vi "PXI-Tasks to Channel Names.vi"(1 "Array":T1[](array[typedef])) -> (0 "Channel Names":string[](array[string]))   [LabVIEW 2020]
uses:
  Type Defs/Task Struct.ctl
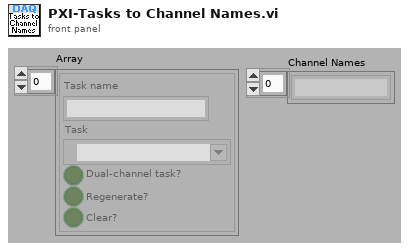
[diagram p1: front panel]
types:
  T1 = typedef "Task Struct.ctl" = cluster{"Task name":string, "Task":refnum<k21>, "Dual-channel task?":bool, "Regenerate?":bool, "Clear?":bool}
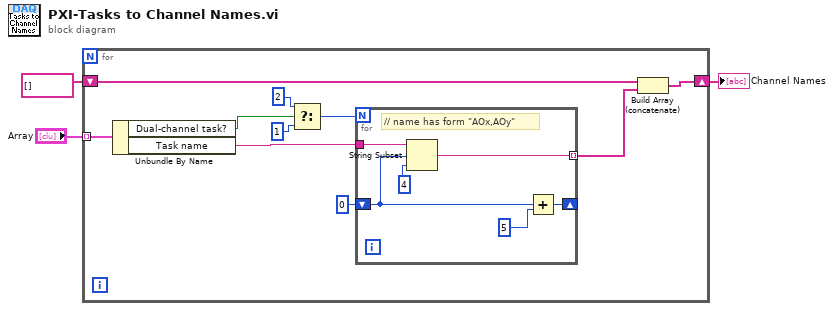
[diagram p0: block diagram]
diagram:
  n1 = for {
    tunnel: "Array" -> [w7] mode=indexing
    shift-right: [w6] -> w1
    shift-left: string[] [] -> [w4]
    n2 = Unbundle By Name(w7) -> ("Dual-channel task?"=w11:bool, "Task name"=w12:string)
    n3 = Select(t=2, s=w11, f=1) -> (s? t:f=w8:i32)
    n4 = for {
      N: w8 -> [_]
      tunnel: w12 -> [w19]
      shift-right: [w17] -> _
      shift-left: 0 -> [w15]
      tunnel: [w14] -> w5 mode=indexing
      # "// name has form \"AOx,AOy\""
      n5 = String Subset(string=w19, offset (0)=w15, length (rest)=4 ("length (rest)")) -> (substring=w14:string)
      n6 = Add(x=w15, y=5) -> (x+y=w17:i32)
    }
    n7 = Build Array (concatenate)(w4, w5) -> (w6:string[])
  }
  "Channel Names" <- w1
